vi "CameraQueryProperties.vi"(8 "error in (no error)":errorcluster, 11 "NIvision in":refnum<class "IMAQdx.lvclass">) -> (0 "error out":errorcluster, 1 "sensor_height":u16, 2 "sensor_width":u16, 3 "NIvision out":refnum<class "IMAQdx.lvclass">, 4 "cam_params":cluster{"String":string, "value":variant}[](array[cluster]) caption="params")   [LabVIEW 2010, in "IMAQdx.lvclass"]
uses:
  IMAQdx.lvclass
  IMAQdx.lvclass/IMAQdx.ctl
  Program Files (x86)/National Instruments/LabVIEW 2010/resource/objmgr/imaqdx.rc
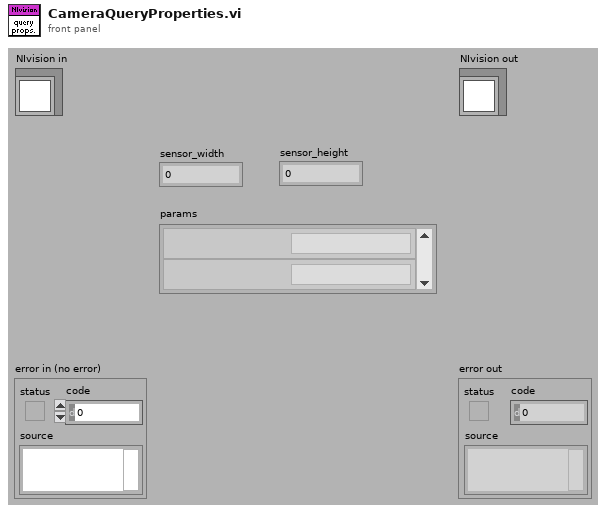
[diagram p1: front panel]
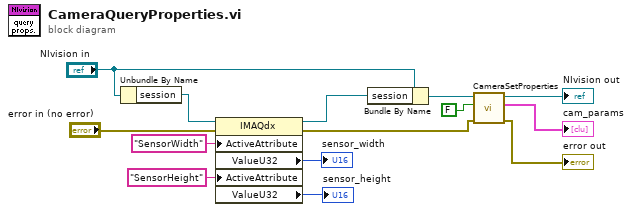
[diagram p0: block diagram]
diagram:
  n1 = Unbundle By Name("NIvision in") -> ("session"=w13:refnum<k21>)
  n2 = property class="IMAQdx"(reference=w13, error in="error in (no error)", "ActiveAttribute"="SensorWidth", "ActiveAttribute"="SensorHeight") -> (reference out=w14:refnum<k21>, error out=w3:errorcluster, "ValueU32"=→"sensor_width":u32, "ValueU32"=→"sensor_height":u32)
  n3 = Bundle By Name(cluster="NIvision in", "session"=w14) -> (w4:refnum<class "IMAQdx.lvclass">)
  n4 = call-dynamic "CameraSetProperties.vi"("error in (no error)"=w3, "set?"=FALSE, "IMAQdx in"=w4) -> ("error out"=→"error out":errorcluster, "cam_params"=→"cam_params":cluster{"String":string, "value":variant}[], "IMAQdx out"=→"NIvision out":refnum<class "IMAQdx.lvclass">)  [unwired: 6 in]
